vi "Four Track to Stereo.vi"(4 "4-Track Audio In":T1) -> (0 "Right Out":dbl[](array[numeric]), 2 "Left Out":dbl[](array[numeric]))   [LabVIEW 2014]
uses:
  Controls/4 Track Audio.ctl
  Controls/Audio In.ctl
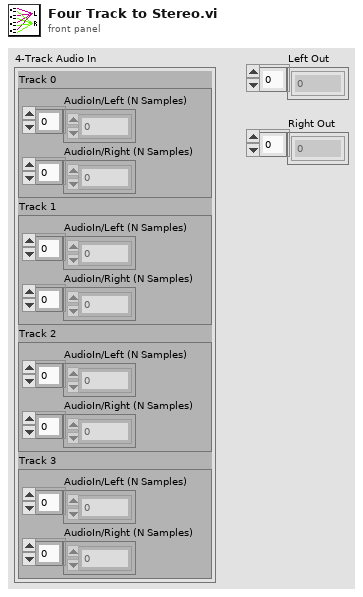
[diagram p1: front panel]
types:
  T1 = typedef "4 Track Audio.ctl" = cluster{"Track 0":T2, "Track 1":T2, "Track 2":T2, "Track 3":T2}
  T2 = typedef "Audio In.ctl" = cluster{"AudioIn/Left (N Samples)":dbl[], "AudioIn/Right (N Samples)":dbl[]}
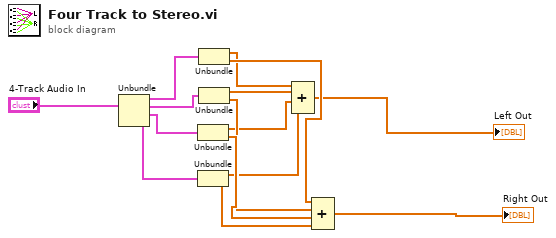
[diagram p0: block diagram]
diagram:
  n1 = Unbundle("4-Track Audio In") -> ("Track 0"=w2:T2, "Track 1"=w3:T2, "Track 2"=w4:T2, "Track 3"=w5:T2)
  n2 = Unbundle(w4) -> ("AudioIn/Left (N Samples)"=w8:dbl[], "AudioIn/Right (N Samples)"=w13:dbl[])
  n3 = Unbundle(w5) -> ("AudioIn/Left (N Samples)"=w9:dbl[], "AudioIn/Right (N Samples)"=w14:dbl[])
  n4 = Unbundle(w2) -> ("AudioIn/Left (N Samples)"=w6:dbl[], "AudioIn/Right (N Samples)"=w11:dbl[])
  n5 = Unbundle(w3) -> ("AudioIn/Left (N Samples)"=w7:dbl[], "AudioIn/Right (N Samples)"=w12:dbl[])
  n6 = Compound Arithmetic op=ADD(w6, w7, w8, w9) -> (→"Left Out":dbl[])
  n7 = Compound Arithmetic op=ADD(w11, w12, w13, w14) -> (→"Right Out":dbl[])
